vi "Turn.vi"(10 "Target":dbl format="%#_13g", 11 "Effort":dbl) -> ()   [LabVIEW 2016]
uses:
  <vilib>/Rock Robotics/WPI/SafetyOutput/WPI_SafetyOutputConfigMenu.ctl
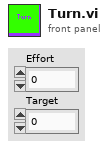
[diagram p1: front panel]
types:
  T1 = typedef "WPI_SafetyOutputConfigMenu.ctl" = enum16{"Enable", "Disable"}
  T2 = typedef "WPI_GyroDevRef.ctl" = cluster{"DevStatus":errorcluster, "Analog Channel":T3, "Offset":dbl, "Gain (VoltsPerDegree/Second)":dbl, "Gyro Type":enum16{"Analog", "XRS450"}, "Handle":i32, "SPI Bus":T4, "Device Found":bool, "Sample Rate":dbl, "Calibrate On Open":bool}
  T3 = typedef "FPGA_AIChannel.ctl" = enum8{"AI 0", "AI 1", "AI 2", "AI 3", "AI MXP 0", "AI MXP 1", "AI MXP 2", "AI MXP 3", "Invalid"}
  T4 = typedef "spi_bus.ctl" = enum16{"SPI On-Board, CS0", "SPI On-Board, CS1", "SPI On-Board, CS2", "SPI On-Board, CS3", "SPI MXP", "Invalid"}
  T5 = typedef "WPI_MotorControlDeviceRef.ctl" = cluster{"DeviceStatus":errorcluster, "Type":T6, "PWM":cluster{"PWM Channel":T7, "DeadBand":T8}, "CAN":cluster{"Device Number":u8, "SetOutput VI Ref":variant, "GetOutput VI Ref":variant, "Enable VI Ref":variant, "Disable VI Ref":variant, "Data":variant}, "Invert":bool}
  T6 = typedef "WPI_MotorControlType.ctl" = enum16{"PWM", "CAN"}
  T7 = typedef "FPGA_DIOPWMChannel.ctl" = enum8{"PWM 0", "PWM 1", "PWM 2", "PWM 3", "PWM 4", "PWM 5", "PWM 6", "PWM 7", "PWM 8", "PWM 9", "PWM MXP 0", "PWM MXP 1", "PWM MXP 2", "PWM MXP 3", "PWM MXP 4", "PWM MXP 5", "PWM MXP 6", "PWM MXP 7", "PWM MXP 8", "PWM MXP 9", "Invalid"}
  T8 = typedef "WPI_PWMDeadband.ctl" = cluster{"Name":string, "maxPositivePwm":i32, "minPositivePwm":i32, "centerPwm":i32, "maxNegativePwm":i32, "minNegativePwm":i32, "angularRange":u16}
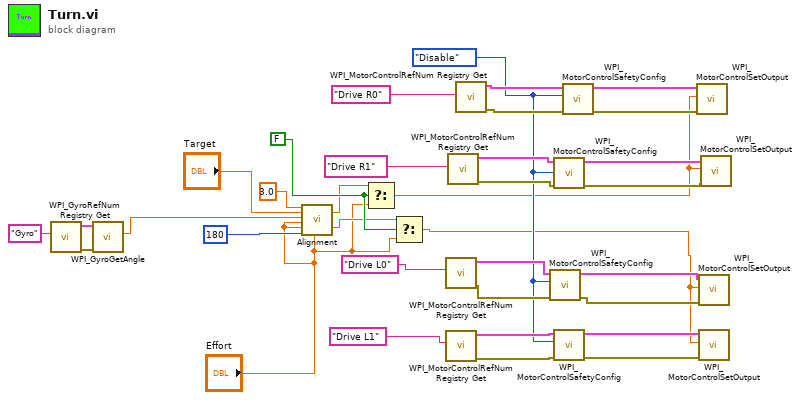
[diagram p0: block diagram]
diagram:
  w6 = FALSE
  w20 = WPI_SafetyOutputConfigMenu."Disable" ("mode")
  n1 = call <vilib>:"WPI_GyroRefNum Registry Get.vi"("refnum name"="Gyro") -> ("error out"=w13:errorcluster, "GyroDevRef"=w12:T2)  [unwired: 9 in]
  n2 = call <vilib>:"WPI_GyroGetAngle.vi"("error in"=w13, "GyroDevRef"=w12) -> ("Angle"=w11:dbl)  [unwired: 5 in, 4 out]
  n3 = call "Alignment.vi"("Range"=3.0, "Target"="Target", "Camera Feedback"=w11, "RightMotorSpeed"="Effort", "LeftMotorSpeed"="Effort", "POV"=180, "Turn_Gain"="Effort") -> ("Right Motor"=w3:dbl, "Left Motor"=w2:dbl)  [unwired: 10 in, 1 out]
  n4 = Select(t=w3, s=w6, f="Effort") -> (s? t:f=w4:dbl)
  n5 = Select(t=w2, s=w6, f="Effort") -> (s? t:f=w5:dbl)
  n6 = call <vilib>:"WPI_MotorControlRefNum Registry Get.vi"("refnum name"="Drive L0") -> ("error out"=w24:errorcluster, "MotorControlDevRef"=w29:T5)  [unwired: 9 in]
  n7 = call <vilib>:"WPI_MotorControlRefNum Registry Get.vi"("refnum name"="Drive L1") -> ("error out"=w23:errorcluster, "MotorControlDevRef"=w27:T5)  [unwired: 9 in]
  n8 = call <vilib>:"WPI_MotorControlRefNum Registry Get.vi"("refnum name"="Drive R1") -> ("error out"=w30:errorcluster, "MotorControlDevRef"=w32:T5)  [unwired: 9 in]
  n9 = call <vilib>:"WPI_MotorControlRefNum Registry Get.vi"("refnum name"="Drive R0") -> ("error out"=w33:errorcluster, "MotorControlDevRef"=w34:T5)  [unwired: 9 in]
  n10 = call <vilib>:"WPI_MotorControlSafetyConfig.vi"("error in (no error)"=w24, "mode"=w20, "MotorControlDevRef"=w29) -> ("error out"=w25:errorcluster, "MotorControlDevRef"=w28:T5)  [unwired: 7 in]
  n11 = call <vilib>:"WPI_MotorControlSafetyConfig.vi"("error in (no error)"=w30, "mode"=w20, "MotorControlDevRef"=w32) -> ("error out"=w19:errorcluster, "MotorControlDevRef"=w31:T5)  [unwired: 7 in]
  n12 = call <vilib>:"WPI_MotorControlSafetyConfig.vi"("error in (no error)"=w23, "mode"=w20, "MotorControlDevRef"=w27) -> ("error out"=w22:errorcluster, "MotorControlDevRef"=w26:T5)  [unwired: 7 in]
  n13 = call <vilib>:"WPI_MotorControlSafetyConfig.vi"("error in (no error)"=w33, "mode"=w20, "MotorControlDevRef"=w34) -> ("error out"=w18:errorcluster, "MotorControlDevRef"=w21:T5)  [unwired: 7 in]
  n14 = call <vilib>:"WPI_MotorControlSetOutput.vi"("error in (no error)"=w18, "Output"=w4, "MotorControlDevRef"=w21) -> ()  [unwired: 6 in, 3 out]
  n15 = call <vilib>:"WPI_MotorControlSetOutput.vi"("error in (no error)"=w25, "Output"=w5, "MotorControlDevRef"=w28) -> ()  [unwired: 6 in, 3 out]
  n16 = call <vilib>:"WPI_MotorControlSetOutput.vi"("error in (no error)"=w22, "Output"=w5, "MotorControlDevRef"=w26) -> ()  [unwired: 6 in, 3 out]
  n17 = call <vilib>:"WPI_MotorControlSetOutput.vi"("error in (no error)"=w19, "Output"=w4, "MotorControlDevRef"=w31) -> ()  [unwired: 6 in, 3 out]
